vi "XYStage.KIM101.GetResource.vi"(8 "error in (no error)":errorcluster, 11 "XYStage.KIM101 in":refnum<class "XYStage.KIM101.lvclass">) -> (0 "error out":errorcluster, 2 "Resource":T1, 3 "XYStage.KIM101 out":refnum<class "XYStage.KIM101.lvclass">)   [LabVIEW 2017, in "XYStage.KIM101.lvclass"]
uses:
  XYStage.KIM101.lvclass
  Typedefs/Resource--Cluster.ctl
  D:/upwork/Laser Measurement Tool/Laser/project/data/Thorlabs.MotionControl.Controls.dll
  data/Thorlabs.MotionControl.Controls.dll
  D:/upwork/Laser Measurement Tool/Laser/project/data/Thorlabs.MotionControl.KCube.InertialMotorCLI.dll
  data/Thorlabs.MotionControl.KCube.InertialMotorCLI.dll
  XYStage.KIM101.lvclass/XYStage.KIM101.ctl
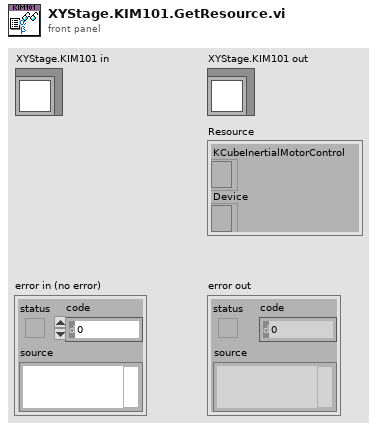
[diagram p1: front panel]
types:
  T1 = typedef "XYStage.KIM101.lvclass/Resource--Cluster.ctl" = cluster{"KCubeInertialMotorControl":refnum<k24>, "Device":refnum<k24>}
  T2 = typedef "XYStage.KIM101.lvclass/PrivateData--Ref.ctl" = refnum<data-value>
  T3 = typedef "XYStage.KIM101.lvclass/PrivateData--Cluster.ctl" = cluster{"Resource":T1}
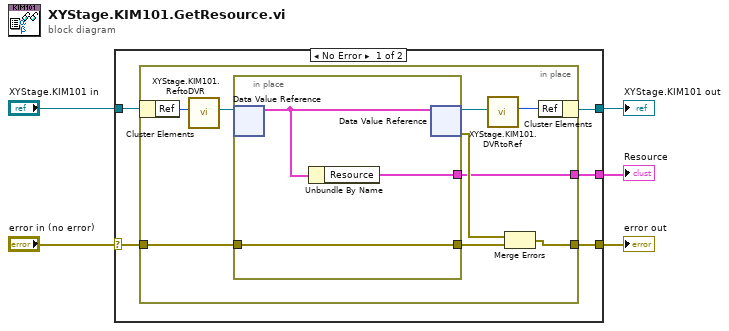
[diagram p0: block diagram]
diagram:
  n1 = case shown="No Error" "error in (no error)" {
    selector: "error in (no error)" -> [w8 w24]
    tunnel: [w7 w24] -> w4
    tunnel: [w9 w23] -> w2
    tunnel: "XYStage.KIM101 in" -> [w10 w23]
    tunnel: [w6 _] -> w1
    frame No Error {
      n2 = in-place {
        in-place-border: w8 -> [w14]
        in-place-border: [w12] -> w7
        in-place-border: [w11] -> w6
        n3 = in-place-cluster #1(w10) -> ("Ref"=w19:u32)
        n4 = call "XYStage.KIM101.ReftoDVR.vi"("Ref"=w19) -> ("Ref"=w17:T2)  [unwired: 10 in]
        n5 = in-place {
          in-place-border: [w22] -> w13
          in-place-border: w14 -> [w22]
          in-place-border: [w20] -> w11
          n6 = in-place-dvr #2(w17) -> (w21:T3)  [unwired: 1 out]
          n7 = Unbundle By Name(w21) -> ("Resource"=w20:T1)
          n8 = in-place-dvr #2(w21) -> (w16:T2, w15:errorcluster)
        }
        n9 = call "XYStage.KIM101.DVRtoRef.vi"("Ref"=w16) -> ("Ref"=w18:u32)  [unwired: 10 in]
        n10 = Merge Errors(w15, w13) -> (w12:errorcluster)
        n11 = in-place-cluster #1("Ref"=w18) -> (w9:refnum<class "XYStage.KIM101.lvclass">)
      }
    }
    frame Error {
    }
  }
  "error out" <- w4
  "XYStage.KIM101 out" <- w2
  "Resource" <- w1
